vi "VisionAim.vi"(8 "Reset PID":bool, 11 "Angle":dbl) -> (2 "In Range":bool, 3 "Turn":dbl)   [LabVIEW 2016]
uses:
  Robot Global Data.vi
panel:
  in  "Latency":i32=7
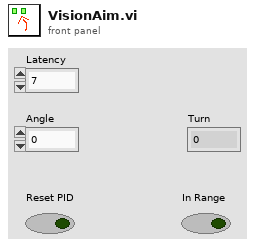
[diagram p1: front panel]
types:
  T1 = cluster{"proportional gain (Kc)":dbl, "integral time (Ti, min)":dbl, "derivative time (Td, min)":dbl}
  T2 = cluster{"theta":dbl, "distance":dbl, "x":dbl, "y":dbl}[]
  T3 = cluster{"theta":dbl, "distance":dbl, "x":dbl, "y":dbl}
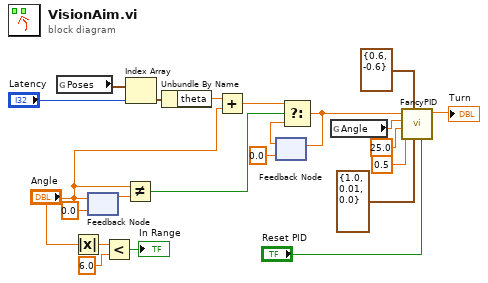
[diagram p0: block diagram]
diagram:
  n1 = global read "Robot Global Data.vi" "Poses"() -> (w22:T2)
  n2 = Absolute Value(x="Angle") -> (abs(x)=w18:dbl)
  n3 = feedback-in #1("Angle") -> ()
  n4 = feedback #1(0.0 ("Angle")) -> (w19:dbl)
  n5 = Less?(x=w18, y=6.0) -> (x < y?=→"In Range":bool)
  n6 = Not Equal?(x="Angle", y=w19) -> (x != y?=w9:bool)
  n7 = Index Array(array=w22, index="Latency") -> (element=w15:T3)
  n8 = Unbundle By Name(w15) -> ("theta"=w14:dbl)
  n9 = Add(x=w14, y="Angle") -> (x+y=w12:dbl)
  n10 = feedback #2(0.0 ("Angle")) -> (w10:dbl)
  n11 = Select(t=w12, s=w9, f=w10) -> (s? t:f=w1:dbl)
  n12 = feedback-in #2(w1) -> ()
  n13 = global read "Robot Global Data.vi" "Angle"() -> (w8:dbl)
  n14 = call "FancyPID.vi"("Reset"="Reset PID", "Gains"=T1 {"proportional gain (Kc)"=1.0, "integral time (Ti, min)"=0.01, "derivative time (Td, min)"=0.0}, "Range"=cluster{"output high":dbl, "output low":dbl} {"output high"=0.6, "output low"=-0.6}, "Disable Range"=0.5, "Integral Range"=25.0, "Process variable"=w8, "Setpoint"=w1) -> ("output"=→"Turn":dbl)  [unwired: 4 in]
